vi "Servicio Basico.vi"(10 "Lista servicios in":string[][](array[string]), 11 "MulticolumnListbox in":refnum<vi>) -> (3 "Lista servicios out":string[][](array[string]))   [LabVIEW 2020, in "Manejador Turnos.lvlib"]
uses:
  Manejador Turnos.lvlib
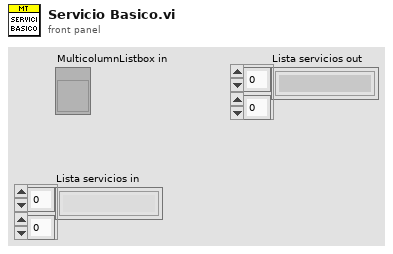
[diagram p1: front panel]
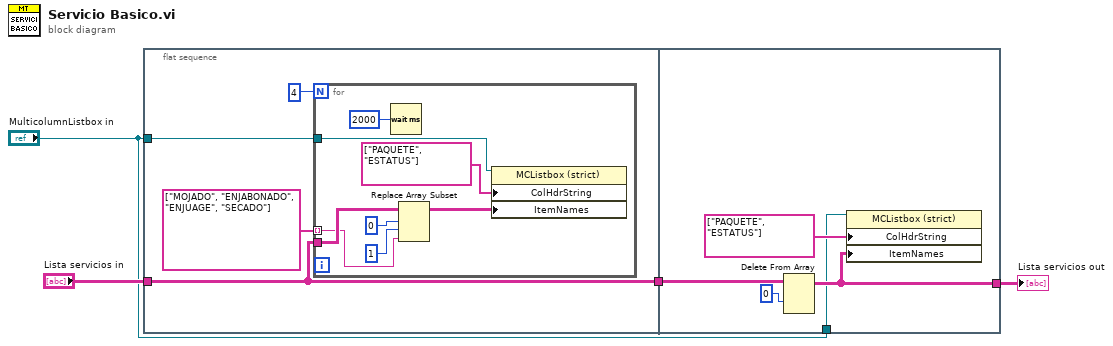
[diagram p0: block diagram]
diagram:
  n1 = flat-sequence {
    tunnel: "Lista servicios in" -> [w6]
    tunnel: [w6] -> w4
    tunnel: "MulticolumnListbox in" -> [w5]
    tunnel: w4 -> [w20]
    tunnel: [w18] -> w3
    tunnel: "MulticolumnListbox in" -> [w17]
    frame #0 {
      n2 = for {
        N: 4 -> [_]
        tunnel: w6 -> [w16]
        tunnel: string[] ["MOJADO", "ENJABONADO", "ENJUAGE", "SECADO"] -> [w13] mode=indexing
        tunnel: w5 -> [w9]
        n3 = Wait (ms)(milliseconds to wait=u32 2000) -> ()  [unwired: 1 out]
        n4 = Replace Array Subset(array=w16, new element=w13, index (row)=0, index (col)=1 ("disabled index (col)")) -> (w10:string[][])
        n5 = property on="Property Node" class="MCListbox (strict)"(reference=w9, "ColHdrString"=string[] ["PAQUETE", "ESTATUS"] ("Column Header Strings[]"), "ItemNames"=w10) -> ()  [unwired: 1 in, 2 out]
      }
    }
    frame #1 {
      n6 = Delete From Array(array=w20, index (row)=0) -> (array with subset deleted=w18:string[][])  [unwired: 2 in, 1 out]
      n7 = property on="Property Node" class="MCListbox (strict)"(reference=w17, "ColHdrString"=string[] ["PAQUETE", "ESTATUS"] ("Column Header Strings[]"), "ItemNames"=w18) -> ()  [unwired: 1 in, 2 out]
    }
  }
  "Lista servicios out" <- w3
